vi "html2image.vi"(6 "size":i64=60000, 7 "IMGPath":path, 8 "Error in":errorcluster caption="Error in (no error)", 11 "html":path=path "") -> (0 "Error out":errorcluster, 3 "IMGPath out":path, 5 "ImagePath":path)   [LabVIEW 2016]
uses:
  <userlib>/_OpenG.lib/array/array.llb/Sort 1D Array (I32)__ogtk.vi
  <userlib>/_OpenG.lib/array/array.llb/Index 1D Array Elements (String)__ogtk.vi
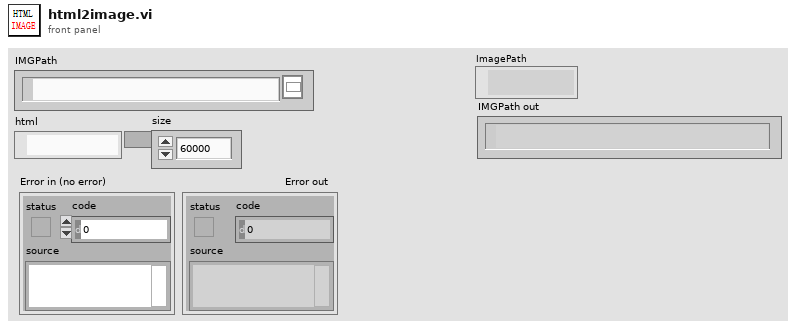
[diagram p1: front panel]
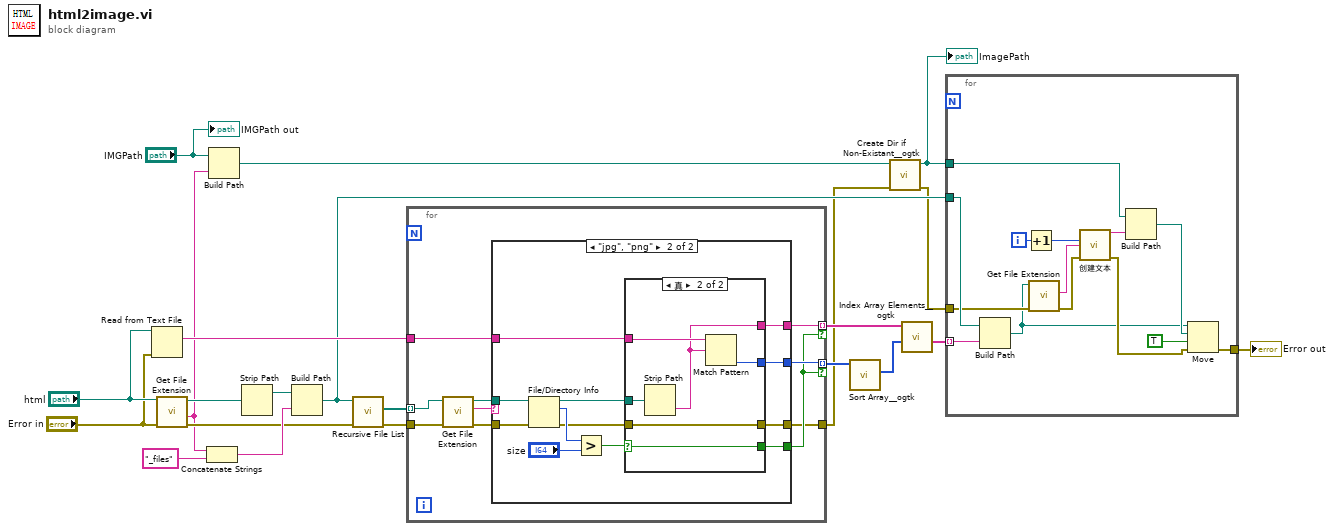
[diagram p0: block diagram]
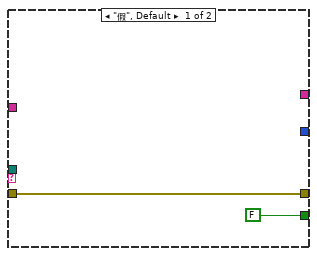
[diagram p2: hidden frame]
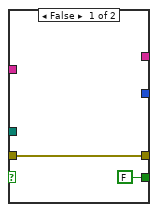
[diagram p3: hidden frame]
diagram:
  n1 = Read from Text File(file (use dialog)="html", error in="Error in") -> (text=w14:string)  [unwired: 2 in, 3 out]
  n2 = call <vilib>:"Get File Extension.vi"("error in (no error)"="Error in", "file"="html") -> ("error out"=w18:errorcluster, "filename without extension"=w10:string, "dup file"=w20:path)  [unwired: 5 in, 2 out]
  n3 = Concatenate Strings(w10, "_files" ("字符串")) -> (w19:string)
  n4 = Build Path(base path="IMGPath", name or relative path=w10) -> (appended path=w8:path)
  n5 = Strip Path(path=w20) -> (stripped path=w21:path)  [unwired: 1 out]
  n6 = Build Path(base path=w21, name or relative path=w19) -> (appended path=w6:path)
  n7 = call <vilib>:"Recursive File List.vi"("error in (no error)"=w18, "Folder Path"=w6) -> ("error out"=w17:errorcluster, "All Files in Dir"=w16:path[])  [unwired: 5 in, 3 out]
  n8 = for {
    tunnel: w17 -> [w32]
    tunnel: w16 -> [w31] mode=indexing
    tunnel: w14 -> [w27]
    tunnel: [w26] -> w13 mode=indexing if=w24
    tunnel: [w25] -> w12 mode=indexing if=w24
    tunnel: [w23] -> w4
    n9 = call <vilib>:"Get File Extension.vi"("error in (no error)"=w32, "file"=w31) -> ("error out"=w30:errorcluster, "lowercase file extension"=w29:string, "dup file"=w28:path)  [unwired: 5 in, 2 out]
    n10 = case shown="\"jpg\", \"png\"" w29 {
      tunnel: w30 -> [w33 w46]
      tunnel: w28 -> [_ w43]
      tunnel: w27 -> [_ w41]
      tunnel: [_ w38] -> w26
      tunnel: [FALSE w37] -> w24
      tunnel: [_ w36] -> w25
      tunnel: [w33 w35] -> w23
      frame "假", Default {
      }
      frame "jpg", "png" {
        n11 = File/Directory Info(path=w43, error in=w46) -> (path out=w40:path, size=w45:i64, error out=w39:errorcluster)  [unwired: 4 out]
        n12 = Greater?(x=w45, y="size") -> (0:w42:bool)
        n13 = case shown="真" w42 {
          selector: w42 -> [_ w51]
          tunnel: w41 -> [_ w53]
          tunnel: w40 -> [_ w54]
          tunnel: w39 -> [w47 w49]
          tunnel: [_ w52] -> w38
          tunnel: [FALSE w51] -> w37
          tunnel: [_ w50] -> w36
          tunnel: [w47 w49] -> w35
          frame False {
          }
          frame True {
            n14 = Strip Path(path=w54) -> (name=w50:string)  [unwired: 1 out]
            n15 = Match Pattern(string=w53, regular expression=w50) -> (offset past match=w52:i32)  [unwired: 1 in, 3 out]
          }
        }
      }
    }
  }
  n16 = call-poly <userlib>:"Sort Array__ogtk.vi"("Array in"=w13) -> ("Sorted Pointers"=w11:i32[])  [unwired: 9 in, 1 out]
  n17 = call <userlib>:"Create Dir if Non-Existant__ogtk.vi"("error in (no error)"=w4, "Directory Path"=w8) -> ("error out"=w3:errorcluster, "dup Directory Path"=w5:path)  [unwired: 7 in, 1 out]
  "ImagePath" <- w5
  n18 = call-poly <userlib>:"Index Array Elements__ogtk.vi"("indices"=w11, "array"=w12) -> ("elements"=w7:string[])  [unwired: 9 in]
  n19 = for {
    tunnel: w7 -> [w67] mode=indexing
    tunnel: w6 -> [w68]
    tunnel: w5 -> [w63]
    tunnel: w3 -> [w61]
    tunnel: [w58] -> w2
    i -> [w66]
    n20 = Build Path(base path=w68, name or relative path=w67) -> (appended path=w56:path)
    n21 = Increment(x=w66) -> (x+1=w55:i32)
    n22 = call <vilib>:"Get File Extension.vi"("error in (no error)"=w61, "file"=w56) -> ("error out"=w60:errorcluster, "lowercase file extension"=w65:string)  [unwired: 5 in, 3 out]
    n23 = call "创建文本"("idx"=w55, "extname"=w65, "error in (no error)"=w60) -> ("Result"=w64:string, "error out"=w59:errorcluster)  [unwired: 11 in]
    n24 = Build Path(base path=w63, name or relative path=w64) -> (appended path=w57:path)
    n25 = Move(source path=w56, error in=w59, 9:TRUE ("覆盖(F)"), 10:w57) -> (error out=w58:errorcluster)  [unwired: 1 in, 2 out]
  }
  "Error out" <- w2
  "IMGPath out" <- "IMGPath"
